vi "test-linear-system-loop-All.vi"(8 "error in (no error)":errorcluster) -> (0 "error out":errorcluster, 3 "ALL TEsts Passed":bool)   [LabVIEW 2019]
panel:
  out "Test 2":bool
  out "Test 1":bool
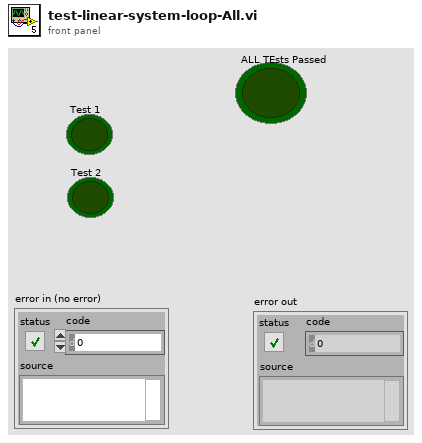
[diagram p1: front panel]
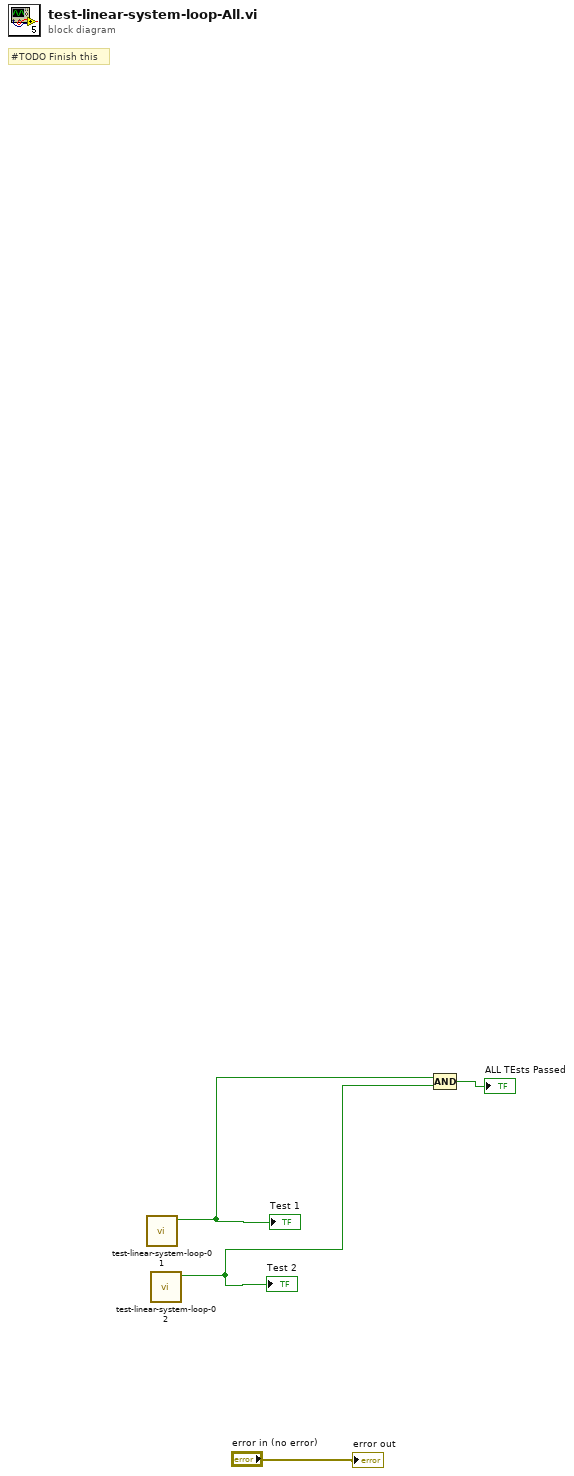
[diagram p0: block diagram]
diagram:
  # "#TODO Finish this"
  n1 = call "test-linear-system-loop-01.vi"() -> ("TEst Passed"=w1:bool)  [unwired: 11 in]
  "Test 1" <- w1
  n2 = call "test-linear-system-loop-02.vi"() -> ("TEst Passed"=w2:bool)  [unwired: 11 in]
  "Test 2" <- w2
  n3 = Compound Arithmetic op=AND(w1, w2) -> (→"ALL TEsts Passed":bool)
  "error out" <- "error in (no error)"
